vi "Main.vi"() -> ()   [LabVIEW 2020]
panel:
  in  "Barcodes in 2":string[](array[string])
  in  "stop 2":bool
  in  "Power Supply \nAddress 2":refnum<visa-resource-name>
  out "Elapsed Time (s)":dbl
  in  "Power Supply \nAddress":refnum<visa-resource-name>
  in  "Barcodes in":string[](array[string])
  out "Individual Tube \nCurrent (Nano Amps)":dbl[](array[numeric])
  out "Test Is Running (Red)\nTest Is Stopped (Green)":bool
  in  "Start":bool
  out "Failed Tubes":string[](array[string])
  out "Actual Voltage Level (V)":dbl format="%#_13g"
  out "Power Supply Trip":bool
  out "Actual Current Limit (nA)":dbl format="%#_13g"
  out "Mesurnment Iteration":i32
  in  "stop":bool
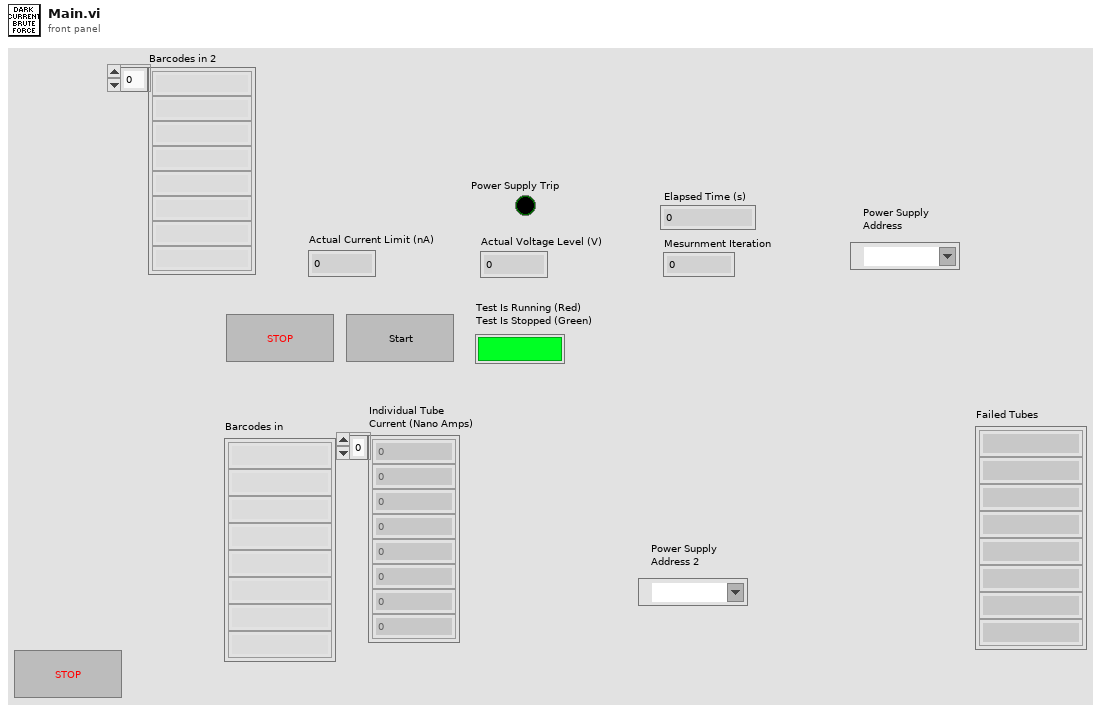
[diagram p1: front panel]
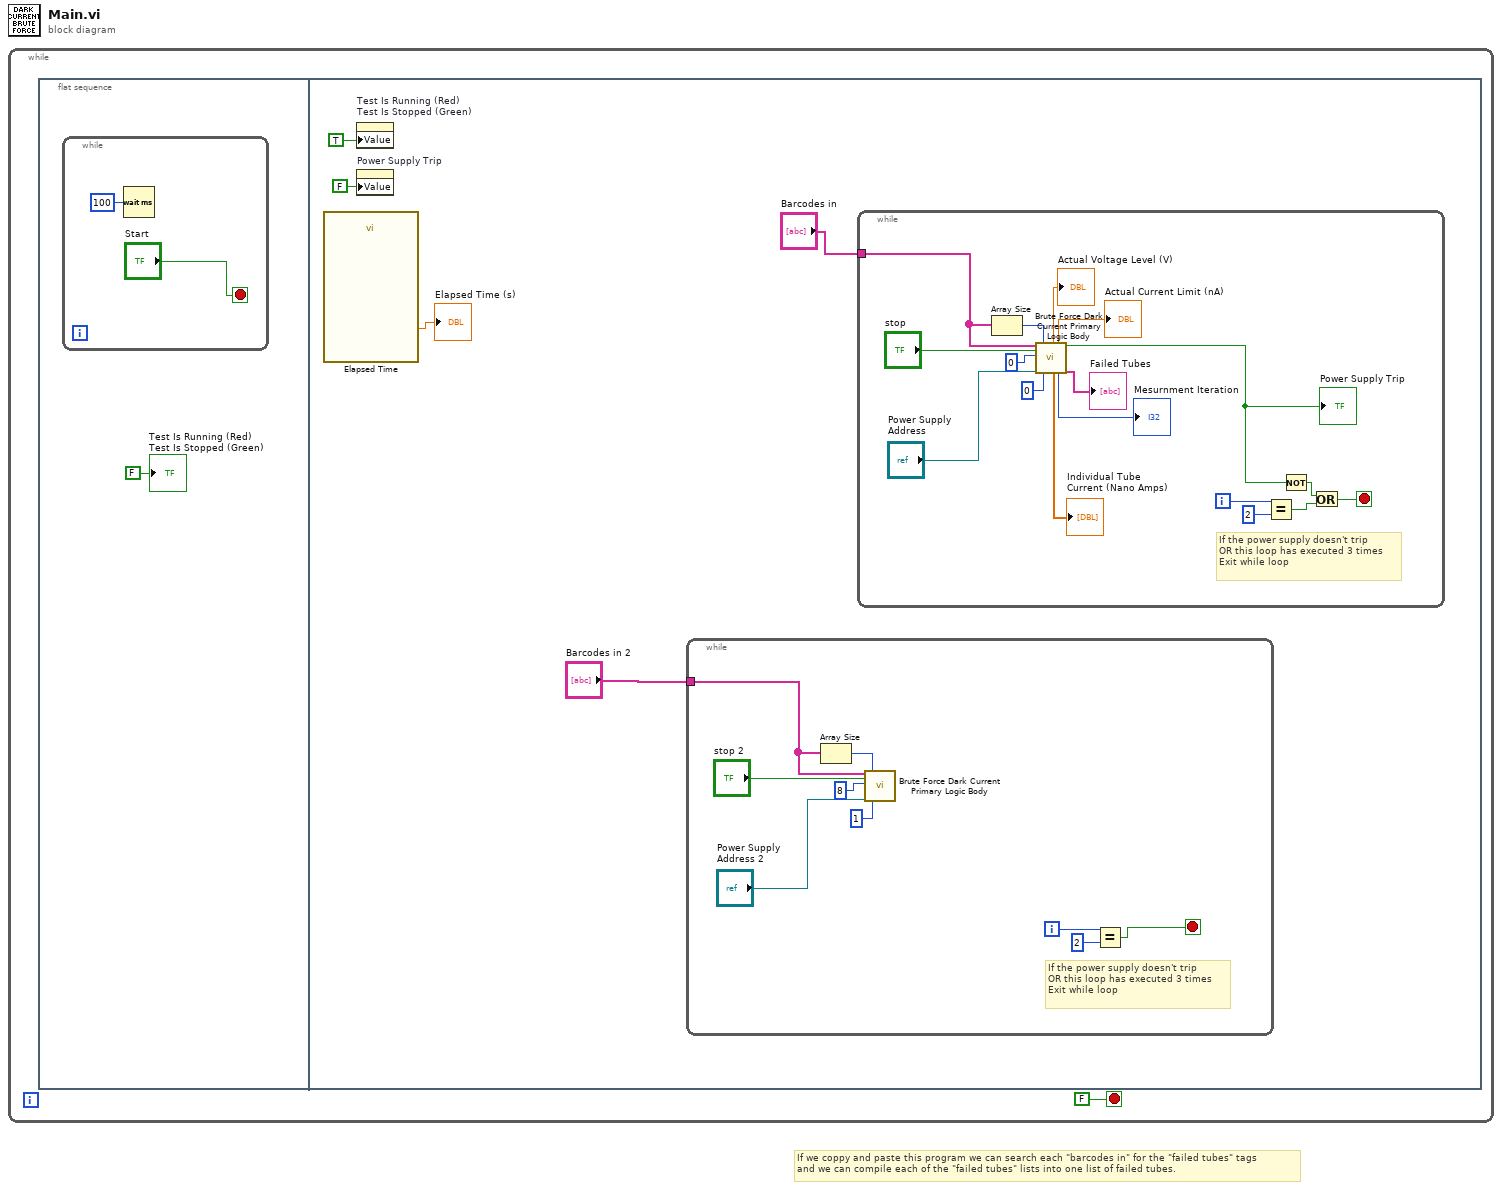
[diagram p0: block diagram]
diagram:
  # "If we coppy and paste this program we can search each \"barcodes in\" for the \"failed tubes\" tags\nand we can compile each of the \"failed tubes\" lists into one list of failed tubes."
  n1 = while {
    stop <- FALSE stop-if-true
    n2 = flat-sequence {
      frame #0 {
        n3 = while {
          stop <- "Start" stop-if-true
          n4 = Wait (ms)(milliseconds to wait=u32 100) -> ()  [unwired: 1 out]
        }
        "Test Is Running (Red)\nTest Is Stopped (Green)" <- FALSE ("Start LED")
      }
      frame #1 {
        n5 = call "Elapsed Time"() -> ("Elapsed Time (s)"=→"Elapsed Time (s)":dbl)  [unwired: 12 in, 7 out]
        n6 = property on="Test Is Running (Red)\nTest Is Stopped (Green)" class="Bool (strict)"("Value"=TRUE) -> ()  [unwired: 2 in, 2 out]
        n7 = property on="Power Supply Trip" class="Bool (strict)"("Value"=FALSE ("Power Supply Trip")) -> ()  [unwired: 2 in, 2 out]
        n8 = while {
          tunnel: "Barcodes in 2" -> [w13]
          i -> [w18]
          stop <- w10 stop-if-true
          # "If the power supply doesn't trip\nOR this loop has executed 3 times Exit while loop"
          n9 = Array Size(array=w13) -> (size(s)=w16:i32)
          n10 = call "Brute Force Dark Current Primary Logic Body.vi"("Barcodes in"=w13, "stop"="stop 2", "First Tube #"=8, "VISA Refnum in"="Power Supply \nAddress 2", "Number of Tubes"=w16, "Channel #"=1) -> ()  [unwired: 8 in, 6 out]
          n11 = Equal?(x=w18, y=2) -> (x = y?=w10:bool)
        }
        n12 = while {
          tunnel: "Barcodes in" -> [w22]
          i -> [w34]
          stop <- w31 stop-if-true
          # "If the power supply doesn't trip\nOR this loop has executed 3 times Exit while loop"
          n13 = Array Size(array=w22) -> (size(s)=w30:i32)
          n14 = call "Brute Force Dark Current Primary Logic Body.vi"("Barcodes in"=w22, "stop"="stop", "First Tube #"=0, "VISA Refnum in"="Power Supply \nAddress", "Number of Tubes"=w30, "Channel #"=0) -> ("Actual Voltage Level (V)"=→"Actual Voltage Level (V)":dbl, "Individual Tube Current (Nano Amps)"=→"Individual Tube \nCurrent (Nano Amps)":dbl[], "Actual Current Limit (nA)"=→"Actual Current Limit (nA)":dbl, "Mesurnment  Iteration"=→"Mesurnment Iteration":i32, "Power Supply Trip"=w20:bool, "Failed Tubes"=→"Failed Tubes":string[])  [unwired: 8 in]
          "Power Supply Trip" <- w20
          n15 = Equal?(x=w34, y=2) -> (x = y?=w32:bool)
          n16 = Not(x=w20) -> (.not. x?=w35:bool)
          n17 = Or(x=w35, y=w32) -> (x .or. y?=w31:bool)
        }
      }
    }
  }
